vi "Initialize Comm (SubVI).vi"(8 "error in (no error)":errorcluster, 11 "Enum":enum16{"TCP", "GPIB"}(ring)) -> (0 "error out":errorcluster, 3 "reference out":refnum<visa-resource-name>)   [LabVIEW 2021]
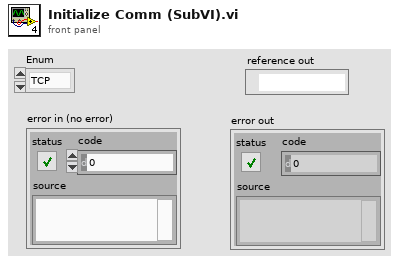
[diagram p1: front panel]
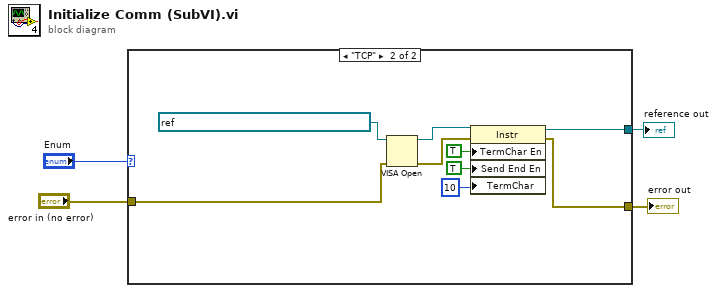
[diagram p0: block diagram]
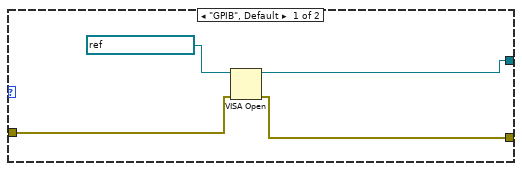
[diagram p2: hidden frame]
diagram:
  n1 = case shown="\"TCP\"" "Enum" {
    tunnel: "error in (no error)" -> [w7 w11]
    tunnel: [w6 w10] -> w3
    tunnel: [w5 w9] -> w2
    frame "GPIB", Default {
      n2 = VISA Open(error in (no error)=w7, VISA resource name=refnum<visa-resource-name> "GPIB1::1::INSTR") -> (VISA resource name=w5:refnum<visa-resource-name>, error out=w6:errorcluster)  [unwired: 3 in]
    }
    frame "TCP" {
      n3 = VISA Open(error in (no error)=w11, VISA resource name=refnum<visa-resource-name> "TCPIP0::192.168.53.1::9878::SOCKET") -> (VISA resource name=w13:refnum<visa-resource-name>, error out=w12:errorcluster)  [unwired: 3 in]
      n4 = property class="Instr"(reference=w13, error in=w12, "TermChar En"=TRUE ("Message Based Settings:Termination Character Enable"), "Send End En"=TRUE ("Message Based Settings:Send End Enable"), "TermChar"=u8 10 ("Message Based Settings:Termination Character")) -> (reference out=w9:refnum<visa-resource-name>, error out=w10:errorcluster)
    }
  }
  "error out" <- w3
  "reference out" <- w2
